vi "Input_Uo_Ulocal_ratio.vi"() -> ()   [LabVIEW 2010]
panel:
  in  "Previous Choice":path
  out "Files Processed":i32(slide) scale=0.0..5.0
  out "Current Filename":path
  in  "stop":bool
  out "Index":i32=22
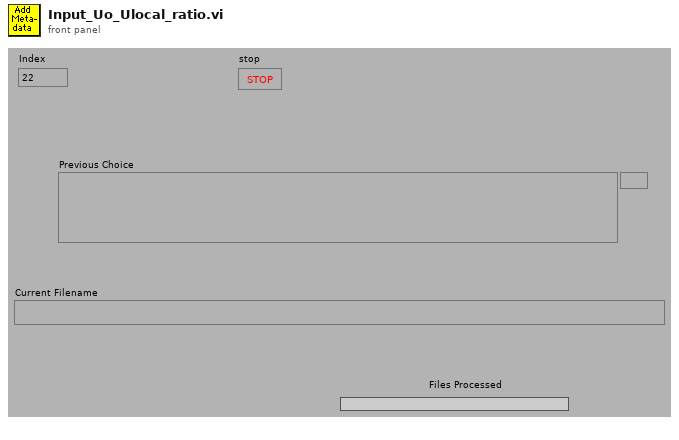
[diagram p1: front panel]
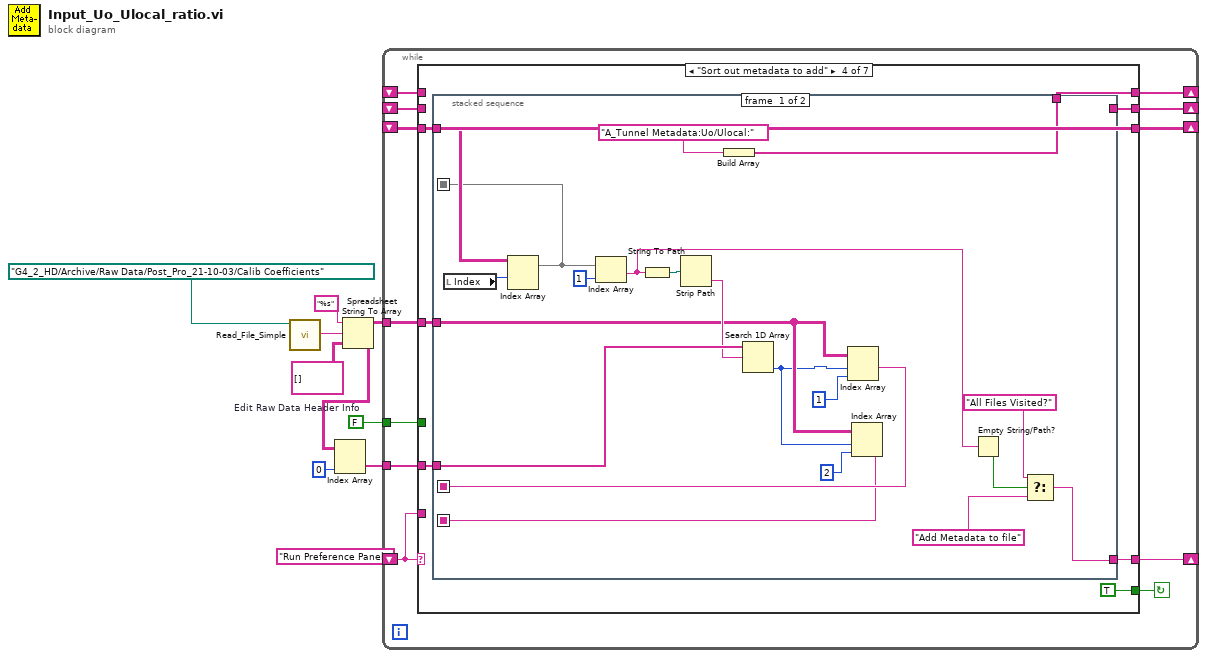
[diagram p0: block diagram]
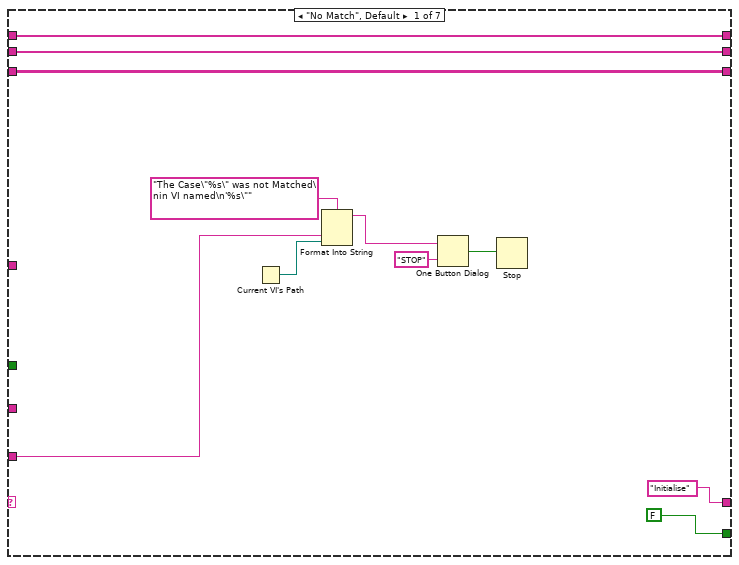
[diagram p2: hidden frame]
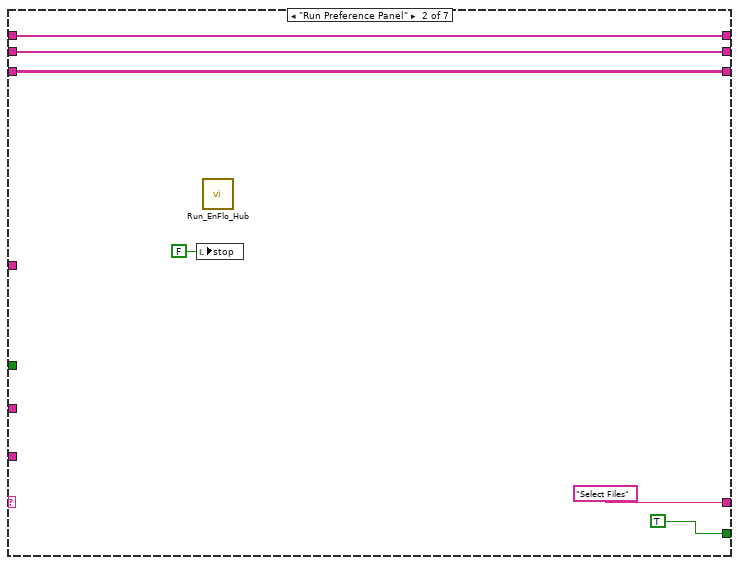
[diagram p3: hidden frame]
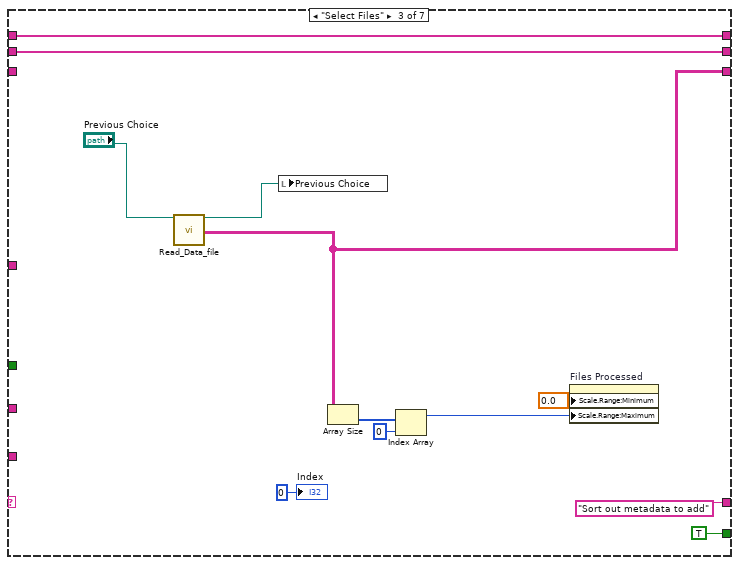
[diagram p4: hidden frame]
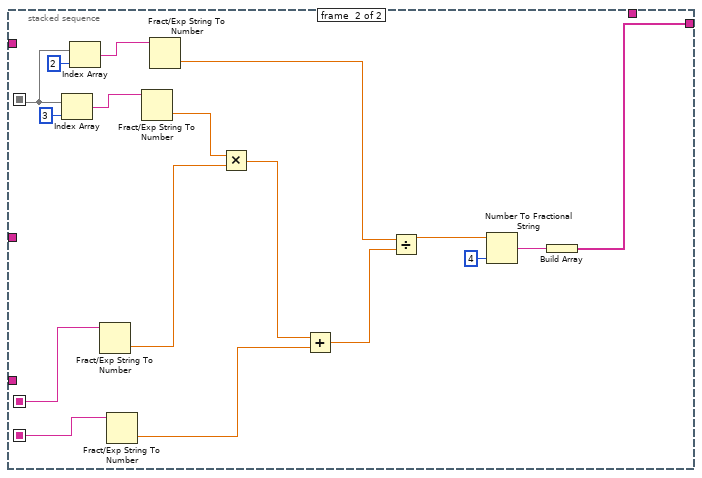
[diagram p5: hidden frame]
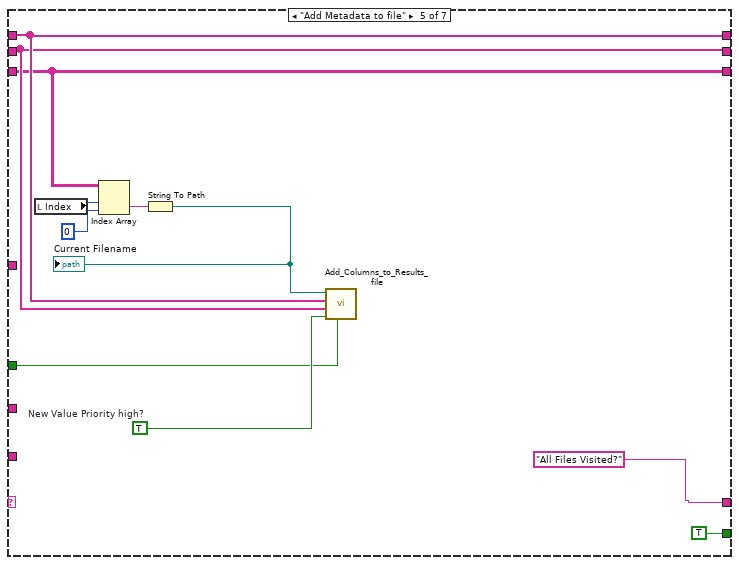
[diagram p6: hidden frame]
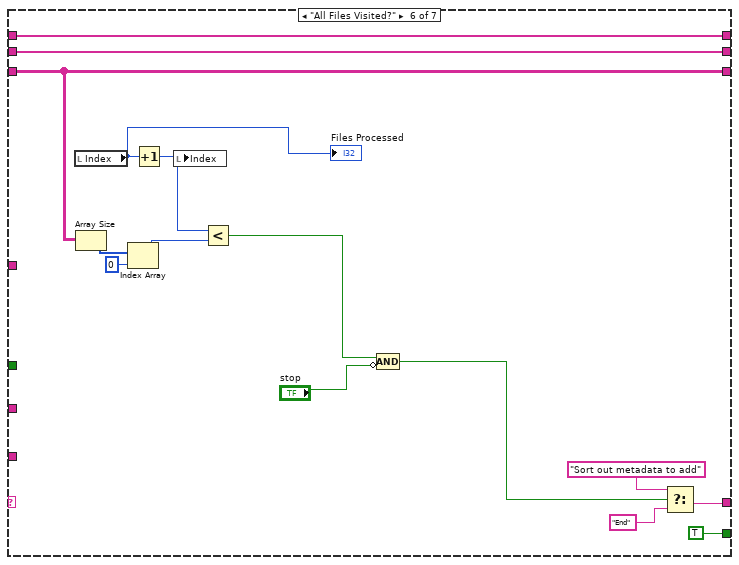
[diagram p7: hidden frame]
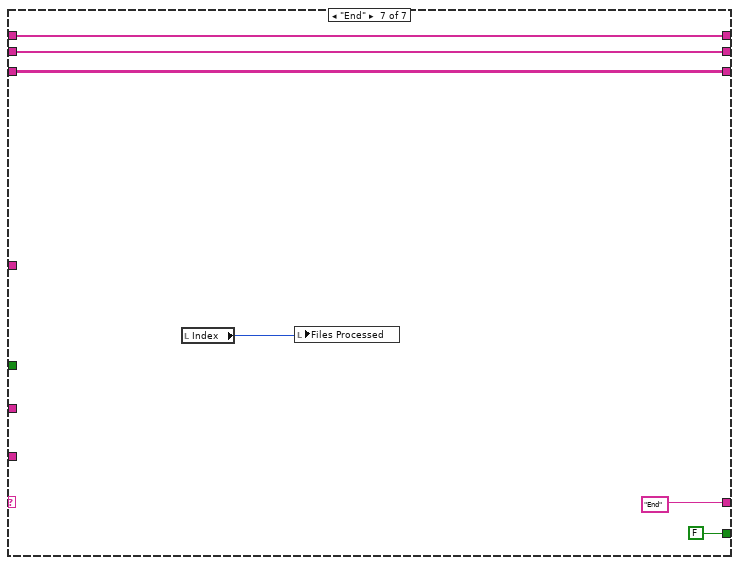
[diagram p8: hidden frame]
diagram:
  w8 = FALSE  # Edit Raw Data Header Info
  n1 = call "Read_File_Simple.vi"("Filename"=path "/G4_2_HD/Archive/Raw Data/Post_Pro_21-10-03/Calib Coefficients" ("Output Filename")) -> ("string"=w2:string)  [unwired: 4 in, 5 out]
  n2 = Spreadsheet String To Array(format string="%s", spreadsheet string=w2, array type (2D Dbl)=string[][] [] ("Channel Values Out")) -> (array=w3:string[][])  [unwired: 1 in]
  n3 = Index Array(array=w3, index (col)=0 ("disabled index (col)")) -> (element=w4:string[])  [unwired: 1 in]
  n4 = while {
    tunnel: w8 -> [w12]
    shift-left: _ -> [w13]
    shift-right: [w14] -> _
    shift-left: _ -> [w16]
    shift-right: [w15] -> _
    shift-left: _ -> [w18]
    shift-right: [w19] -> _
    shift-left: "Run Preference Panel" -> [w20]
    shift-right: [w21] -> _
    tunnel: w4 -> [w11]
    tunnel: w3 -> [w10]
    stop <- w17 continue-if-true
    n5 = case shown="\"Sort out metadata to add\"" w20 {
      tunnel: [FALSE TRUE TRUE TRUE TRUE TRUE FALSE] -> w17
      tunnel: ["Initialise" "Select Files" "Sort out metadata to add" w54 "All Files Visited?" w109 "End"] -> w21
      tunnel: w20 -> [w27 _ _ _ _ _ _]
      tunnel: [w24 w37 w42 w55 w98 w120 w123] -> w19
      tunnel: w18 -> [w24 w37 _ w55 w98 w120 w123]
      tunnel: w16 -> [w23 w35 w48 _ w101 w116 w126]
      tunnel: [w23 w35 w48 w56 w101 w116 w126] -> w15
      tunnel: [w22 w34 w49 w51 w100 w115 w125] -> w14
      tunnel: w13 -> [w22 w34 w49 _ w100 w115 w125]
      tunnel: w12 -> [_ _ _ _ w99 _ _]
      tunnel: w11 -> [_ _ _ w53 _ _ _]
      tunnel: w10 -> [_ _ _ w52 _ _ _]
      frame "No Match", Default {
        n6 = Current VI's Path() -> (path=w26:path)
        n7 = Format Into String(format string="The Case\"%s\" was not Matched\nin VI named\n'%s\"" ("Format String"), w27, w26) -> (resulting string=w30:string)  [unwired: 2 in, 1 out]
        n8 = One Button Dialog(message=w30, button name ("OK")="STOP") -> (true=w28:bool)
        n9 = Stop(stop? (T)=w28) -> ()
      }
      frame "Run Preference Panel" {
        n10 = local write "stop"(FALSE ("stop")) -> ()
        n11 = call "Run_EnFlo_Hub.vi"() -> ()  [unwired: 8 in]
      }
      frame "Select Files" {
        n12 = call "Read_Data_file.vi"("Results file"="Previous Choice") -> ("Results file Out"=w43:path, "Channel Values Out"=w42:string[][])  [unwired: 9 in, 8 out]
        n13 = local write "Previous Choice"(w43) -> ()
        n14 = Array Size(array=w42) -> (size(s)=w41:i32[])
        n15 = Index Array(array=w41, index=0) -> (element=w40:i32)
        n16 = property on="Files Processed" class="Slide (strict)"("Scale.Range:Minimum"=0.0, "Scale.Range:Maximum"=w40) -> ()  [unwired: 2 in, 2 out]
        "Index" <- 0 ("Index")
      }
      frame "Sort out metadata to add" {
        n17 = stacked-sequence {
          seq-local: [w68 _] -> [_ w94]
          seq-local: [w65 _] -> [_ w93]
          seq-local: [w63 _] -> [_ w84]
          tunnel: [w75 _] -> w56
          tunnel: w55 -> [w74 _]
          tunnel: [w59 _] -> w54
          tunnel: w53 -> [w71 _]
          tunnel: w52 -> [w66 _]
          tunnel: [_ w78] -> w51
          frame #0 {
            n18 = local read "Index"() -> (w77:i32)
            n19 = Index Array(array=w74, index (row)=w77) -> (element=w63:string[])  [unwired: 1 in]
            n20 = Index Array(array=w63, index=1) -> (element=w62:string)
            n21 = String To Path(string=w62) -> (path=w72:path)
            n22 = Strip Path(path=w72) -> (name=w70:string)  [unwired: 1 out]
            n23 = Build Array("A_Tunnel Metadata:Uo/Ulocal:") -> (w75:string[])
            n24 = Search 1D Array(1D array=w71, element=w70) -> (index of element=w64:i32)  [unwired: 1 in]
            n25 = Index Array(array=w66, index (row)=w64, index (col)=1 ("disabled index (col)")) -> (element=w68:string)
            n26 = Index Array(array=w66, index (row)=w64, index (col)=2 ("disabled index (col)")) -> (element=w65:string)
            n27 = Empty String/Path?(string/path=w62) -> (empty?=w61:bool)
            n28 = Select(t="All Files Visited?", s=w61, f="Add Metadata to file") -> (s? t:f=w59:string)
          }
          frame #1 {
            n29 = Index Array(array=w84, index=3) -> (element=w91:string)
            n30 = Index Array(array=w84, index=2) -> (element=w86:string)
            n31 = Fract/Exp String To Number(string=w94) -> (number=w89:dbl)  [unwired: 3 in, 1 out]
            n32 = Fract/Exp String To Number(string=w93) -> (number=w87:dbl)  [unwired: 3 in, 1 out]
            n33 = Fract/Exp String To Number(string=w91) -> (number=w90:dbl)  [unwired: 3 in, 1 out]
            n34 = Fract/Exp String To Number(string=w86) -> (number=w83:dbl)  [unwired: 3 in, 1 out]
            n35 = Multiply(x=w90, y=w89) -> (x*y=w88:dbl)
            n36 = Add(x=w88, y=w87) -> (x+y=w82:dbl)
            n37 = Divide(x=w83, y=w82) -> (x/y=w81:dbl)
            n38 = Number To Fractional String(number=w81, precision (6)=i16 4) -> (F-format string=w79:string)  [unwired: 2 in]
            n39 = Build Array(w79) -> (w78:string[])
          }
        }
      }
      frame "Add Metadata to file" {
        w102 = TRUE  # New Value Priority high?
        n40 = local read "Index"() -> (w103:i32)
        n41 = Index Array(array=w98, index (row)=w103, index (col)=0 ("disabled index (col)")) -> (element=w104:string)
        n42 = String To Path(string=w104) -> (path=w95:path)
        "Current Filename" <- w95
        n43 = call "Add_Columns_to_Results_file.vi"("Edit Raw Data Header Info"=w99, "New Value Priority high?"=w102, "New Values In"=w100, "New Chs In"=w101, "Data filename"=w95) -> ()  [unwired: 5 out]
      }
      frame "All Files Visited?" {
        n44 = local read "Index"() -> (w114:i32)
        "Files Processed" <- w114
        n45 = Array Size(array=w120) -> (size(s)=w108:i32[])
        n46 = Index Array(array=w108, index=0) -> (element=w106:i32)
        n47 = Increment(x=w114) -> (x+1=w119:i32)
        n48 = local write "Index"(w119) -> ()
        n49 = Less?(x=w119, y=w106) -> (x < y?=w117:bool)
        n50 = Compound Arithmetic op=AND(w117, invert "stop") -> (w112:bool)
        n51 = Select(t="Sort out metadata to add", s=w112, f="End") -> (s? t:f=w109:string)
      }
      frame "End" {
        n52 = local read "Index"() -> (w121:i32)
        n53 = local write "Files Processed"(w121) -> ()
      }
    }
  }
